vi "manuele bediening.vi"(0 "voorwaarts":bool, 5 "achterwaarts":bool, 7 "rechts draaien achteruit":bool, 9 "links draaien":bool, 12 "rechts draaien":bool, 13 "manuele bediening":bool, 14 "links draaien achteruit":bool) -> ()   [LabVIEW 2019]
uses:
  <vilib>/myRIO/Common/Instrument Driver Framework/Utilities/typedefs/Analog Scaling Constants.ctl
  <vilib>/myRIO/Common/Instrument Driver Framework/Utilities/typedefs/Analog Scaling Constants List.ctl
  <vilib>/myRIO/Common/Instrument Driver Framework/myRIO v1.0/AO/typedefs/AO Channels Enum.ctl
  <vilib>/myRIO/Common/Instrument Driver Framework/myRIO v1.0/AO/typedefs/AO Channels List.ctl
  <vilib>/myRIO/Common/Instrument Driver Framework/Utilities/typedefs/Generic FPGA Reference.ctl
  <vilib>/myRIO/Common/Instrument Driver Framework/Utilities/typedefs/myRIO v1.0 Reference.ctl
  <vilib>/myRIO/Common/Instrument Driver Framework/Utilities/typedefs/Hardware Version Enum.ctl
  <vilib>/myRIO/Common/Instrument Driver Framework/Utilities/typedefs/myRIO Generic Hardware Reference.ctl
  <vilib>/myRIO/Instrument Drivers/Onboard IO/AO/typedefs/AO Reference.ctl
  <vilib>/myRIO/Instrument Drivers/Onboard IO/AO/AO.lvlib
  <vilib>/myRIO/Instrument Drivers/Onboard IO/AO/vis/Write.vi
  <vilib>/userDefined/High Color/nirio_resource_hc.ctl
  <vilib>/myRIO/Common/Instrument Driver Framework/myRIO v1.0/AO/vis/myRIO v1.1 Open AO.vi
  <vilib>/myRIO/Instrument Drivers/Onboard IO/AO/vis/myRIO AO Open.xnode
  <vilib>/myRIO/Common/Instrument Driver Framework/Utilities/vis/Is FPGA Ref Available.vi
  <vilib>/myRIO/Express VI/Onboard IO/AO/AO Express VI.xnode
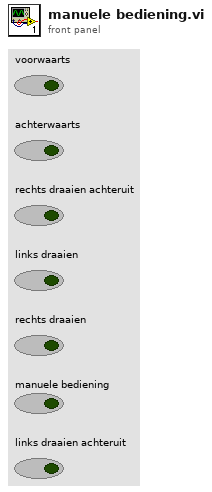
[diagram p1: front panel]
types:
  T1 = typedef "AO.lvlib/AO Reference.ctl" = cluster{"myRIO Reference":T2, "AO Channel List":T6, "AO Scaling Constant List":T8}
  T2 = typedef "myRIO Generic Hardware Reference.ctl" = cluster{"myRIO Model":T3, "myRIO Hardware Reference":T4}
  T3 = typedef "Hardware Version Enum.ctl" = enum16{"Unknown", "myRIO-1900", "myRIO-1950", "roboRIO", "NI ELVIS RIO CM", "ELVIS III"}
  T4 = typedef "myRIO v1.0 Reference.ctl" = cluster{"Generic FPGA Reference":T5, "Allow multiple opens":bool}
  T5 = typedef "Generic FPGA Reference.ctl" = refnum<k20>
  T6 = typedef "AO Channels List.ctl" = T7[]
  T7 = typedef "AO Channels Enum.ctl" = enum16{"Not Connected", "AudioOut/Left", "AudioOut/Right", "C/AO0", "C/AO1", "A/AO0", "A/AO1", "B/AO0", "B/AO1"}
  T8 = typedef "Analog Scaling Constants List.ctl" = T9[]
  T9 = typedef "Analog Scaling Constants.ctl" = cluster{"LSB Weight (Volts)":dbl, "Offset (Volts)":dbl, "Signed?":bool}
  T10 = typedef "nirio_resource_hc.ctl" = tag
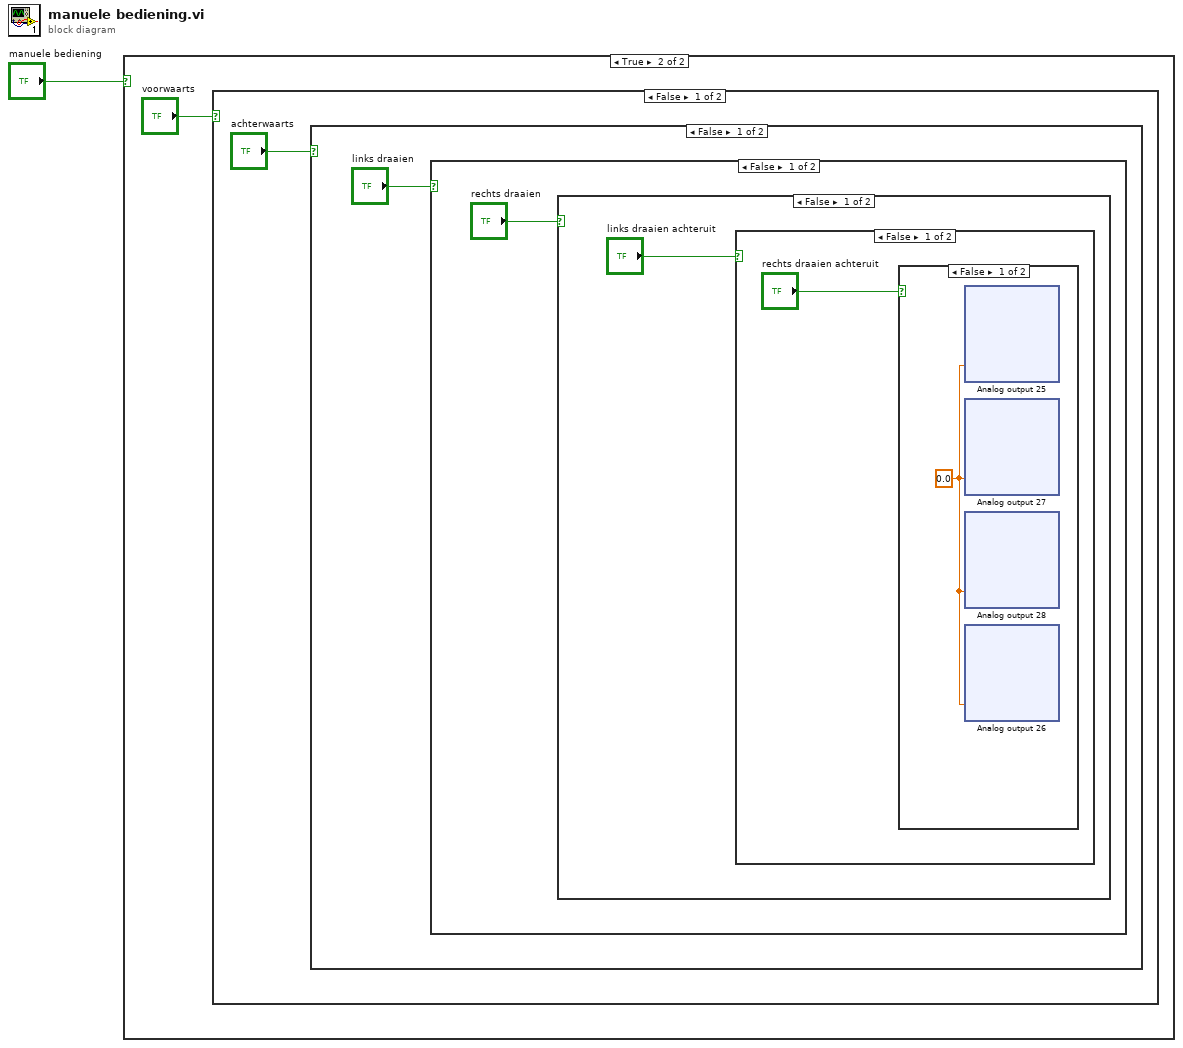
[diagram p0: block diagram]
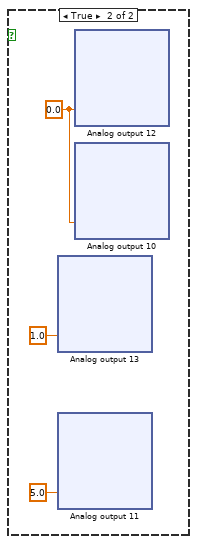
[diagram p3: hidden frame]
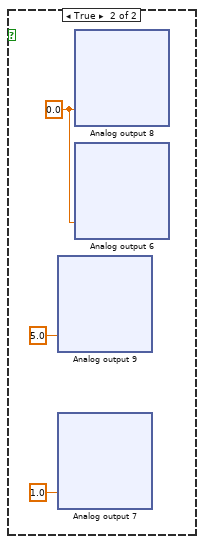
[diagram p4: hidden frame]
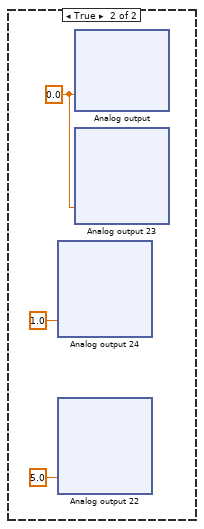
[diagram p5: hidden frame]
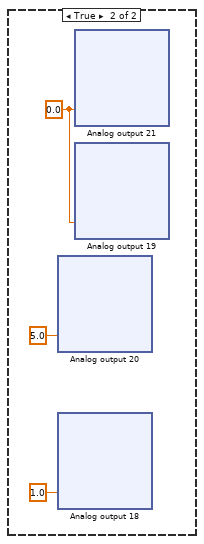
[diagram p6: hidden frame]
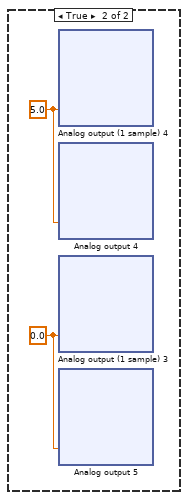
[diagram p7: hidden frame]
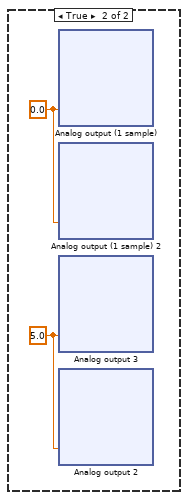
[diagram p8: hidden frame]
diagram:
  n1 = case shown="True" "manuele bediening" {
    frame False {
    }
    frame True {
      n2 = case shown="False" "voorwaarts" {
        frame False {
          n3 = case shown="False" "achterwaarts" {
            frame False {
              n4 = case shown="False" "links draaien" {
                frame False {
                  n5 = case shown="False" "rechts draaien" {
                    frame False {
                      n6 = case shown="False" "links draaien achteruit" {
                        frame False {
                          n7 = case shown="False" "rechts draaien achteruit" {
                            frame False {
                              w8 = 0.0
                              n8 = xnode "Analog output 25"("A/AO0 (Pin 2)"=w8) -> ()  [unwired: 1 in, 1 out]
                              n9 = xnode "Analog output 27"("B/AO0 (Pin 2)"=w8) -> ()  [unwired: 1 in, 1 out]
                              n10 = xnode "Analog output 28"("B/AO1 (Pin 4)"=w8) -> ()  [unwired: 1 in, 1 out]
                              n11 = xnode "Analog output 26"("A/AO1 (Pin 4)"=w8) -> ()  [unwired: 1 in, 1 out]
                            }
                            frame True {
                              w158 = 0.0
                              n12 = xnode "Analog output 13"("A/AO0 (Pin 2)"=1.0) -> ()  [unwired: 1 in, 1 out]
                              n13 = xnode "Analog output 11"("B/AO0 (Pin 2)"=5.0) -> ()  [unwired: 1 in, 1 out]
                              n14 = xnode "Analog output 12"("A/AO1 (Pin 4)"=w158) -> ()  [unwired: 1 in, 1 out]
                              n15 = xnode "Analog output 10"("B/AO1 (Pin 4)"=w158) -> ()  [unwired: 1 in, 1 out]
                            }
                          }
                        }
                        frame True {
                          w308 = 0.0
                          n16 = xnode "Analog output 9"("A/AO0 (Pin 2)"=5.0) -> ()  [unwired: 1 in, 1 out]
                          n17 = xnode "Analog output 7"("B/AO0 (Pin 2)"=1.0) -> ()  [unwired: 1 in, 1 out]
                          n18 = xnode "Analog output 8"("A/AO1 (Pin 4)"=w308) -> ()  [unwired: 1 in, 1 out]
                          n19 = xnode "Analog output 6"("B/AO1 (Pin 4)"=w308) -> ()  [unwired: 1 in, 1 out]
                        }
                      }
                    }
                    frame True {
                      w461 = 0.0
                      n20 = xnode "Analog output 24"("A/AO1 (Pin 4)"=1.0) -> ()  [unwired: 1 in, 1 out]
                      n21 = xnode "Analog output 22"("B/AO1 (Pin 4)"=5.0) -> ()  [unwired: 1 in, 1 out]
                      n22 = xnode "Analog output"("A/AO0 (Pin 2)"=w461) -> ()  [unwired: 1 in, 1 out]
                      n23 = xnode "Analog output 23"("B/AO0 (Pin 2)"=w461) -> ()  [unwired: 1 in, 1 out]
                    }
                  }
                }
                frame True {
                  w612 = 0.0
                  n24 = xnode "Analog output 20"("A/AO1 (Pin 4)"=5.0) -> ()  [unwired: 1 in, 1 out]
                  n25 = xnode "Analog output 18"("B/AO1 (Pin 4)"=1.0) -> ()  [unwired: 1 in, 1 out]
                  n26 = xnode "Analog output 21"("A/AO0 (Pin 2)"=w612) -> ()  [unwired: 1 in, 1 out]
                  n27 = xnode "Analog output 19"("B/AO0 (Pin 2)"=w612) -> ()  [unwired: 1 in, 1 out]
                }
              }
            }
            frame True {
              w761 = 5.0
              w762 = 0.0
              n28 = xnode "Analog output (1 sample) 4"("A/AO0 (Pin 2)"=w761) -> ()  [unwired: 1 in, 1 out]
              n29 = xnode "Analog output 4"("B/AO0 (Pin 2)"=w761) -> ()  [unwired: 1 in, 1 out]
              n30 = xnode "Analog output (1 sample) 3"("A/AO1 (Pin 4)"=w762) -> ()  [unwired: 1 in, 1 out]
              n31 = xnode "Analog output 5"("B/AO1 (Pin 4)"=w762) -> ()  [unwired: 1 in, 1 out]
            }
          }
        }
        frame True {
          w911 = 5.0
          w912 = 0.0
          n32 = xnode "Analog output (1 sample)"("B/AO0 (Pin 2)"=w912) -> ()  [unwired: 1 in, 1 out]
          n33 = xnode "Analog output (1 sample) 2"("A/AO0 (Pin 2)"=w912) -> ()  [unwired: 1 in, 1 out]
          n34 = xnode "Analog output 3"("A/AO1 (Pin 4)"=w911) -> ()  [unwired: 1 in, 1 out]
          n35 = xnode "Analog output 2"("B/AO1 (Pin 4)"=w911) -> ()  [unwired: 1 in, 1 out]
        }
      }
    }
  }
